vi "DCA Convert Stimulus Cluster.vi"(4 "Conversion":enum16{"Cluster - HTML", "HTML - Cluster"}(ring), 6 "Stimulus Key Array In":T2, 7 "Stimulus Cluster In":T1={"Use Instrument"=FALSE, "Normalize"=FALSE, "Blank Screen"=FALSE, "Measurement Type"=enum."Diode", "Range"=enum."Auto", "Resolution"=enum."Auto"}) -> (1 "Stimulus Cluster Out":T1={"Use Instrument"=FALSE, "Normalize"=FALSE, "Blank Screen"=FALSE, "Measurement Type"=enum."Diode", "Range"=enum."Auto", "Resolution"=enum."Auto"}, 2 "Stumulus HTML Out":string)   [LabVIEW 2011]
uses:
  ITK EXT/utils/keyedarr.llb/Keyed Array.ctl
  TypeDefs/DCA Stimulus Parameters.ctl
  ITK EXT/utils/strutil.llb/Case Matching.ctl
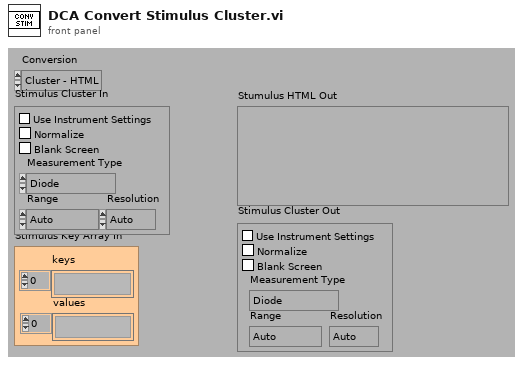
[diagram p1: front panel]
types:
  T1 = typedef "DCA Stimulus Parameters.ctl" = cluster{"Use Instrument":bool, "Normalize":bool, "Blank Screen":bool, "Measurement Type":enum16{"Voltage DC", "Voltage DC Ratio", "Voltage AC", "Current DC", "Current AC", "Resistance", "Fresistance", "Frequency", "Period", "Continuity", "Diode"}, "Range":enum16{"Auto", "Minimum", "Maximum", "100", "1,000", "10,000", "100,000", "1,000,000", "10,000,000", "100,000,000"}, "Resolution":enum16{"Auto", "4 1/2", "5 1/2", "6 1/2"}}
  T2 = typedef "Keyed Array.ctl" = cluster{"keys":string[], "values":string[]}
  T3 = enum16{"Auto", "Minimum", "Maximum", "100", "1,000", "10,000", "100,000", "1,000,000", "10,000,000", "100,000,000"}
  T4 = typedef "Case Matching.ctl" = enum16{"a != A", "a == A", "system"}
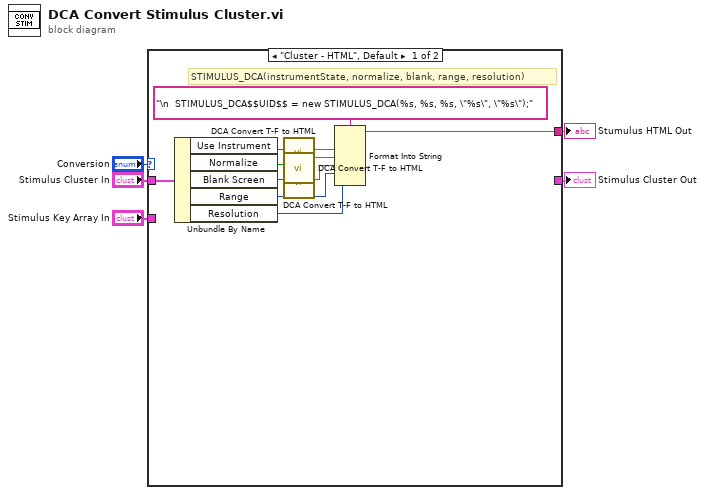
[diagram p0: block diagram]
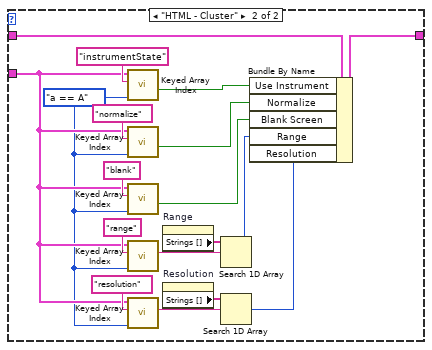
[diagram p2: hidden frame]
diagram:
  n1 = case shown="\"Cluster - HTML\", Default" "Conversion" {
    tunnel: "Stimulus Cluster In" -> [w16 w34]
    tunnel: "Stimulus Key Array In" -> [_ w27]
    tunnel: [w14 _] -> w2
    tunnel: [_ w33] -> w1
    frame "Cluster - HTML", Default {
      # "STIMULUS_DCA(instrumentState, normalize, blank, range, resolution)"
      n2 = Unbundle By Name(w16) -> ("Use Instrument"=w10:bool, "Normalize"=w13:bool, "Blank Screen"=w8:bool, "Range"=w11:T3, "Resolution"=w6:enum16{"Auto", "4 1/2", "5 1/2", "6 1/2"})
      n3 = call "DCA Convert T-F to HTML.vi"("(T/F)"=w10) -> ("HTML (true/false)"=w9:string)  [unwired: 10 out]
      n4 = call "DCA Convert T-F to HTML.vi"("(T/F)"=w13) -> ("HTML (true/false)"=w12:string)  [unwired: 10 out]
      n5 = call "DCA Convert T-F to HTML.vi"("(T/F)"=w8) -> ("HTML (true/false)"=w7:string)  [unwired: 10 out]
      n6 = Format Into String(format string="\n  STIMULUS_DCA$$UID$$ = new STIMULUS_DCA(%s, %s, %s, \"%s\", \"%s\");", w9, w12, w7, w11, w6) -> (resulting string=w14:string)  [unwired: 2 in, 1 out]
    }
    frame "HTML - Cluster" {
      w17 = Case_Matching."a == A" ("case matching (sensitive)")
      n7 = call "Keyed Array Index.vi"("case matching (sensitive)"=w17, "key"="instrumentState", "array in"=w27) -> ("valid key"=w18:bool)  [unwired: 1 in, 3 out]
      n8 = call "Keyed Array Index.vi"("case matching (sensitive)"=w17, "key"="normalize", "array in"=w27) -> ("valid key"=w19:bool)  [unwired: 1 in, 3 out]
      n9 = call "Keyed Array Index.vi"("case matching (sensitive)"=w17, "key"="blank", "array in"=w27) -> ("valid key"=w20:bool)  [unwired: 1 in, 3 out]
      n10 = call "Keyed Array Index.vi"("case matching (sensitive)"=w17, "key"="range", "array in"=w27) -> ("value"=w25:string)  [unwired: 1 in, 3 out]
      n11 = call "Keyed Array Index.vi"("case matching (sensitive)"=w17, "key"="resolution", "array in"=w27) -> ("value"=w26:string)  [unwired: 1 in, 3 out]
      n12 = property on="Range" class="Enum (strict)"() -> ("Strings []"=w22:string[])  [unwired: 2 in, 2 out]
      n13 = property on="Resolution" class="Enum (strict)"() -> ("Strings []"=w21:string[])  [unwired: 2 in, 2 out]
      n14 = Search 1D Array(1D array=w22, element=w25) -> (index of element=w24:i32)  [unwired: 1 out]
      n15 = Search 1D Array(1D array=w21, element=w26) -> (index of element=w23:i32)  [unwired: 1 out]
      n16 = Bundle By Name(cluster=w34, "Use Instrument"=w18, "Normalize"=w19, "Blank Screen"=w20, "Range"=w24, "Resolution"=w23) -> (w33:T1)
    }
  }
  "Stumulus HTML Out" <- w2
  "Stimulus Cluster Out" <- w1
